vi "Wegzähler.vi"(8 "error in (no error)":errorcluster caption="Fehler (Eingang, kein Fehler)", 9 "letzter Wert":dbl, 11 "aktueller Wert":dbl) -> (0 "error out":errorcluster caption="Fehler (Ausgang)")   [LabVIEW 2014]
panel:
  # "Ermittelt den Differenzbetrag des zurückgelegten Weges und addiert zur globalen Variable Wegzähler"
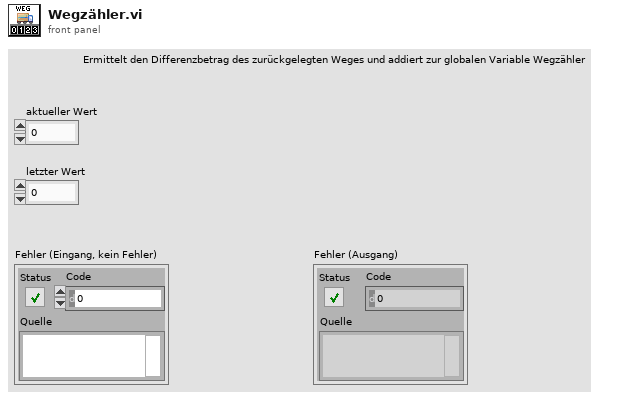
[diagram p1: front panel]
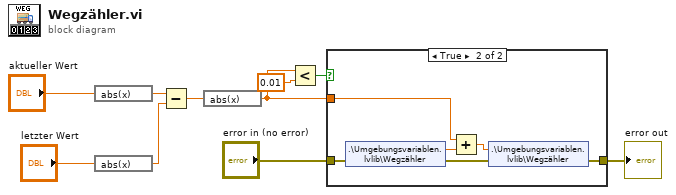
[diagram p0: block diagram]
diagram:
  n1 = expression code="abs(x)"("aktueller Wert") -> (w10:dbl)
  n2 = expression code="abs(x)"("letzter Wert") -> (w9:dbl)
  n3 = Subtract(x=w10, y=w9) -> (x-y=w4:dbl)
  n4 = expression code="abs(x)"(w4) -> (w3:dbl)
  n5 = Less?(x=w3, y=0.01) -> (x < y?=w2:bool)
  n6 = case shown="True" w2 {
    tunnel: "error in (no error)" -> [w11 w15]
    tunnel: [w11 w13] -> w5
    tunnel: w3 -> [_ w12]
    frame False {
    }
    frame True {
      n7 = shared-variable ".\\Umgebungsvariablen.lvlib\\Wegzähler"(error in=w15) -> (w17:dbl, error out=w14:errorcluster)
      n8 = Add(x=w12, y=w17) -> (x+y=w16:dbl)
      n9 = shared-variable ".\\Umgebungsvariablen.lvlib\\Wegzähler"(w16, error in=w14) -> (error out=w13:errorcluster)
    }
  }
  "error out" <- w5
